vi "CIGrab.vi"(8 "Camera data":variant, 9 "TrackingParameters":T1={"Corner-based bead pos (out)"=[], "QTrk Instance"={"QTrk Pointer"=0}, "Tracking Config"={"Number of steps"=0, "ZLUT stepsize (um)"=0.0, "Z correction factor"=0.0, "Start piezo Z (um)"=0.0, "Pixel size (nm)"=0.0, "2D Localization Type"=enum."Quadrant Interpolation", "Z Command (None)"=enum."Nothing"}, "ResultManager"={"InstancePtr"=0}, "Send to queue?"=TRUE}, 10 "Output Queue":refnum<queue>, 11 "GrabControlQueue":refnum<queue>) -> (0 "Camera (out)":variant)   [LabVIEW 2011]
uses:
  BeadTracker2.llb/CmdData_NewFrame.ctl
  <vilib>/vision/Image Controls.llb/IMAQ Image.ctl
  BeadTracker2.llb/CmdEnum_CameraFrameType.ctl
  BeadTracker2.llb/CIGrabParams.ctl
  qtrk/QTrk.llb/QTrkInstance.ctl
  BeadTracker2.llb/TrackingConfigType.ctl
  qtrk/QTrk.llb/QTrkLocalizationType.ctl
  qtrk/QTrk.llb/QTrkZCommandType.ctl
  qtrk/QTrk.llb/ResultManagerInstance.ctl
  BeadTracker2.llb/CIGrabControlMsg.ctl
  BeadTracker2.llb/CIGrabControlMsgEnum.ctl
  mkCameraData.ctl
  CameraConfig.ctl
  BeadTracker2.llb/GenericCameraConfigType.ctl
panel:
  in  "Check ROIs":bool
  out "Status Information : Lost Frames":u32
  in  "Tracking enabled?":bool
  in  "stop":bool
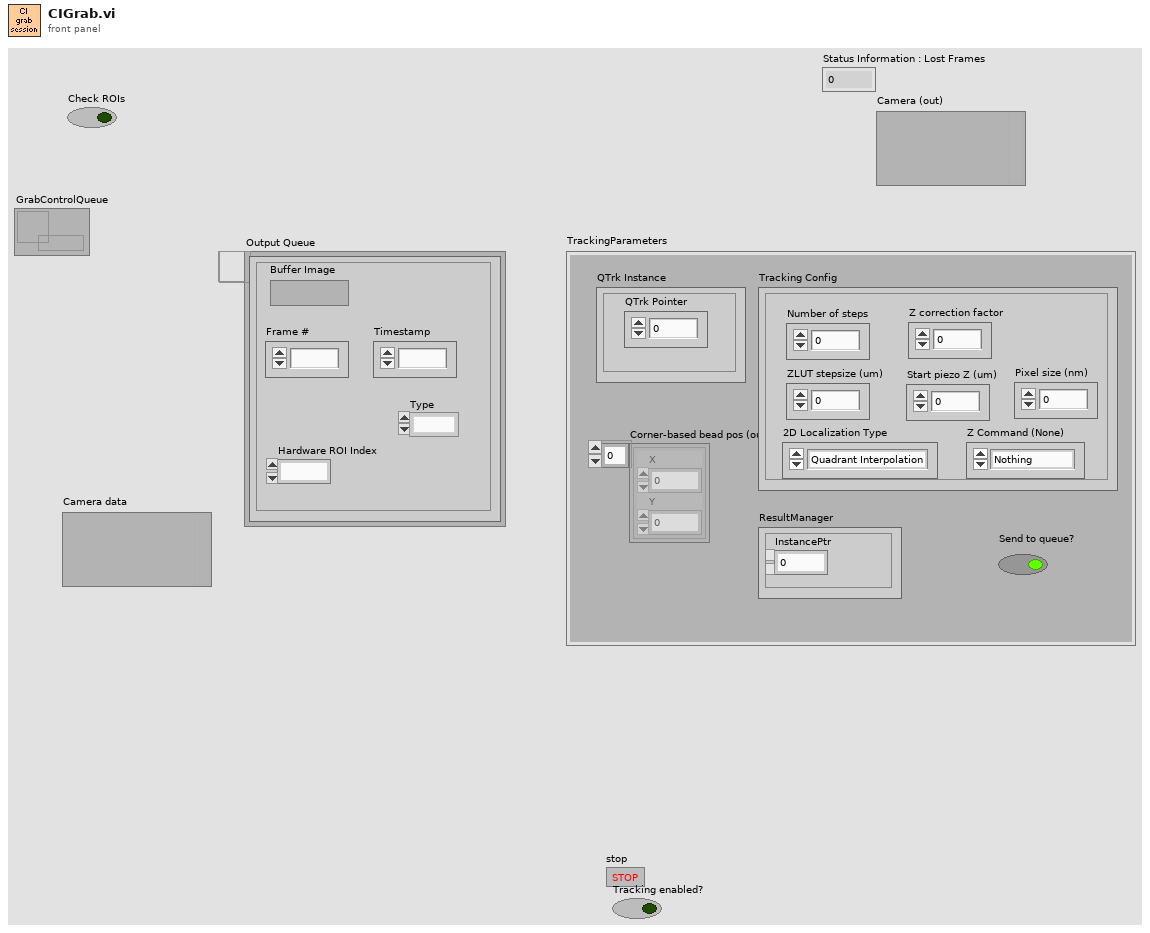
[diagram p1: front panel]
types:
  T1 = typedef "CIGrabParams.ctl" = cluster{"Corner-based bead pos (out)":cluster{"X":i32, "Y":i32}[], "QTrk Instance":T2, "Tracking Config":T3, "ResultManager":T6, "Send to queue?":bool}
  T2 = typedef "QTrkInstance.ctl" = cluster{"QTrk Pointer":u64}
  T3 = typedef "TrackingConfigType.ctl" = cluster{"Number of steps":i32, "ZLUT stepsize (um)":sgl, "Z correction factor":sgl, "Start piezo Z (um)":sgl, "Pixel size (nm)":sgl, "2D Localization Type":T4, "Z Command (None)":T5}
  T4 = typedef "QTrkLocalizationType.ctl" = enum16{"Center-of-Mass", "1D Cross-Correlation", "Quadrant Interpolation", "Gaussian 2D MLE"}
  T5 = typedef "QTrkZCommandType.ctl" = enum16{"Nothing", "ComputeZ", "BuildRadialZLUT", "BuildImageZLUT", "RadialZLUT+ImageZLUT"}
  T6 = typedef "ResultManagerInstance.ctl" = cluster{"InstancePtr":u64}
  T7 = typedef "mkCameraData.ctl" = cluster{"Session":refnum<k11>, "Settings":T8}
  T8 = typedef "CameraConfig.ctl" = cluster{"Gain [1-4]":sgl, "Offset":i16, "Mode":i16, "ROIs":cluster{"X":i32, "Y":i32}[], "ROI Size":cluster{"X":i32, "Y":i32}, "Number of buffers":i32, "Use hardware multiple-ROI?":bool, "GenericCameraConfig":T9}
  T9 = typedef "GenericCameraConfigType.ctl" = cluster{"Framerate (Hz)":i32, "Exposure time (us)":i32, "Image size":cluster{"Width":i32, "Height":i32}}
  T10 = typedef "QTrkComputedSettings.ctl" = cluster{"QTrk Settings":T11, "Derived settings":cluster{"ZLUT Radial Steps":i32, "ZLUT Angular Steps":i32, "ZLUT Max Radius":sgl, "QI Radial Steps":i32, "QI Angular Steps\nPer Quadrant":i32, "QI Max Radius":sgl}}
  T11 = typedef "QTrkSettings.ctl" = cluster{"Image width":i32, "Image height":i32, "Number of threads (CPU based)":i32, "CUDA Device":i32, "COM Background correction factor":sgl, "ZLUT MinRadius":sgl, "ZLUT Radial sample density":sgl, "ZLUT Angular sample density":sgl, "ZLUT ROI Coverage":sgl, "QI Iterations":i32, "QI MinRadius":sgl, "QI Radial sample density":sgl, "QI Angular sample density":sgl, "QI ROI Coverage":sgl, "QI Angular Step \nIteration Factor":sgl, "XCOR Profile Length":i32, "XCOR Profile Width":i32, "XCOR Iterations":i32, "Gaussian 2D Fit Iterations":i32, "Gaussian 2D Sigma (pixels)":sgl}
  T12 = typedef "CIGrabControlMsg.ctl" = cluster{"Msg":T13}
  T13 = typedef "CIGrabControlMsgEnum.ctl" = enum16{"Stop", "EnableTracking", "DisableTracking"}
  T14 = typedef "CmdEnum_CameraFrameType.ctl" = enum16{"Full", "HardwareROI", "EndGrabMarker"}
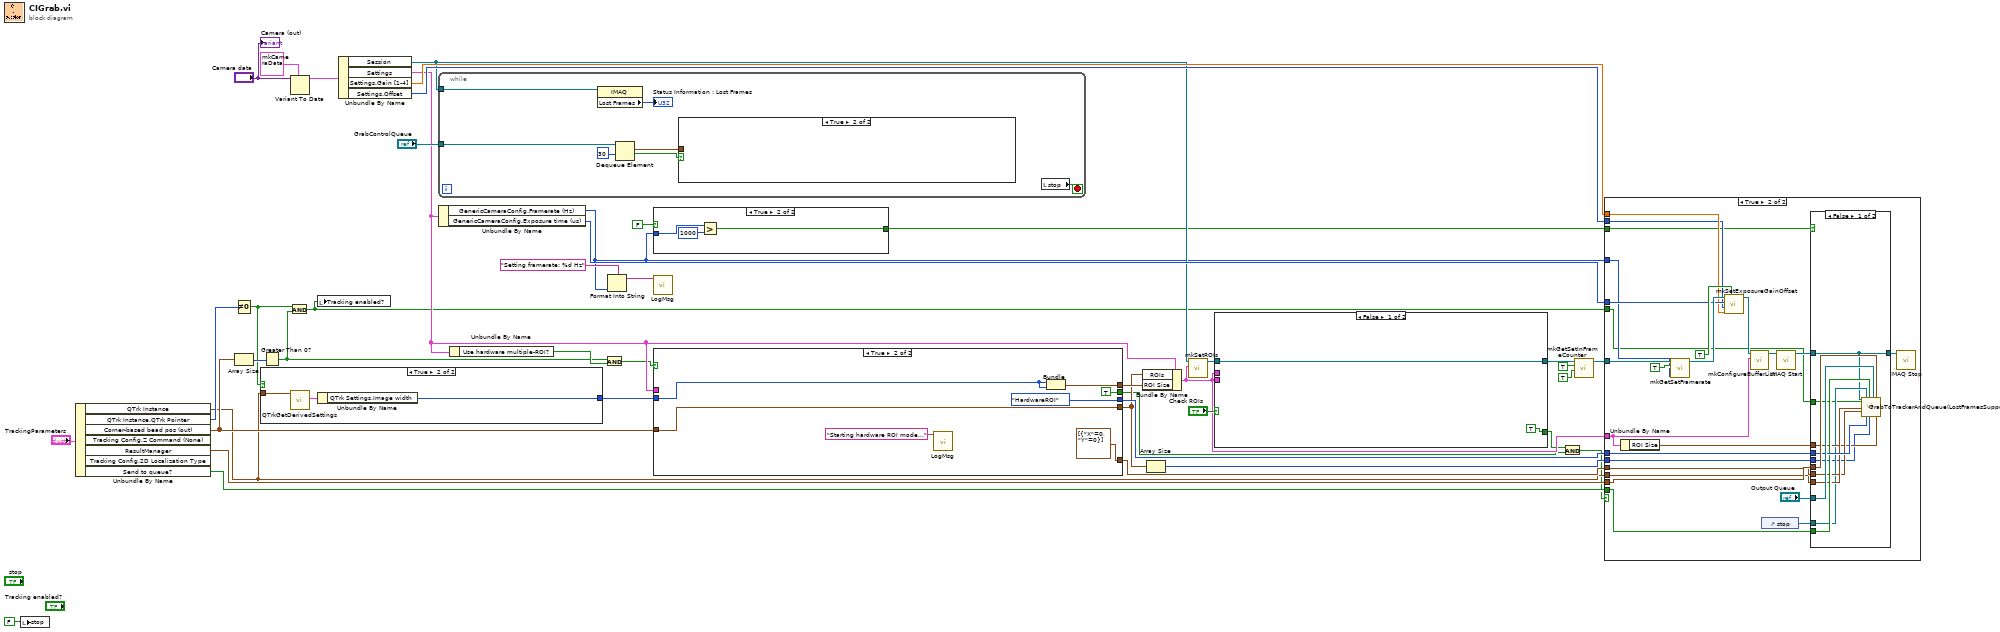
[diagram p0: block diagram]
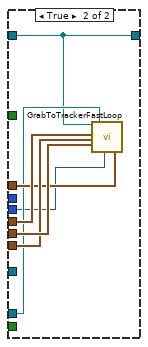
[diagram p3: hidden frame]
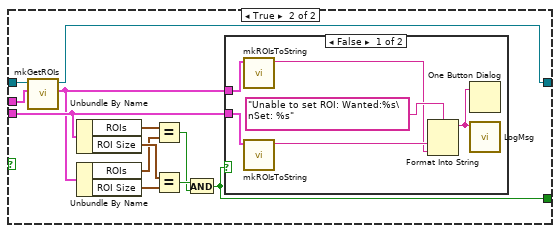
[diagram p4: hidden frame]
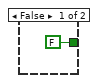
[diagram p6: hidden frame]
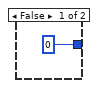
[diagram p7: hidden frame]
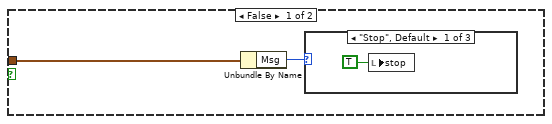
[diagram p8: hidden frame]
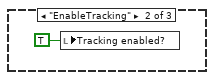
[diagram p9: hidden frame]
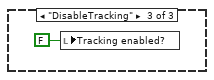
[diagram p10: hidden frame]
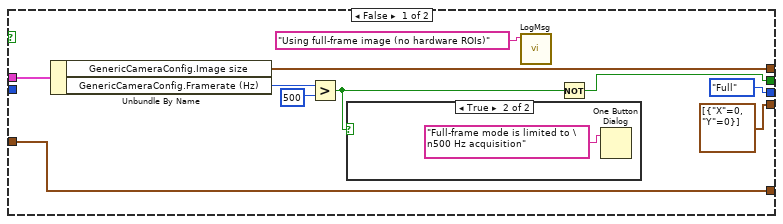
[diagram p11: hidden frame]
diagram:
  n1 = local write "stop"(FALSE ("stop")) -> ()
  n2 = Unbundle By Name("TrackingParameters") -> ("QTrk Instance"=w15:T2, "QTrk Instance.QTrk Pointer"=w37:u64, "Corner-based bead pos (out)"=w31:cluster{"X":i32, "Y":i32}[], "ResultManager"=w35:T6, "Send to queue?"=w27:bool)  [unwired: 2 out]
  n3 = Not Equal To 0?(x=w37) -> (x != 0?=w16:bool)
  n4 = Array Size(array=w31) -> (size(s)=w30:i32)
  n5 = case shown="True" w16 {
    tunnel: w15 -> [_ w46]
    tunnel: [0 ("Image width") w45] -> w14
    frame False {
    }
    frame True {
      n6 = call "QTrkGetDerivedSettings.vi"("QTrk Instance"=w46) -> ("Derived settings"=w47:T10)  [unwired: 5 in, 5 out]
      n7 = Unbundle By Name(w47) -> ("QTrk Settings.Image width"=w45:i32)
    }
  }
  n8 = Greater Than 0?(x=w30) -> (x > 0?=w28:bool)
  n9 = Variant To Data(type=T7 {"Session"=refnum, "Settings"={"Gain [1-4]"=1.0, "Offset"=50, "Mode"=6, "ROIs"=[], "ROI Size"={"X"=0, "Y"=0}, "Number of buffers"=40, "Use hardware multiple-ROI?"=FALSE, "GenericCameraConfig"={"Framerate (Hz)"=0, "Exposure time (us)"=0, "Image size"={"Width"=0, "Height"=0}}}} ("Camera data"), Variant="Camera data") -> (data=w8:T7)  [unwired: 1 in, 1 out]
  n10 = And(x=w16, y=w28) -> (x .and. y?=w10:bool)
  n11 = local write "Tracking enabled?"(w10) -> ()
  n12 = Unbundle By Name(w8) -> ("Session"=w26:refnum<k11>, "Settings"=w22:T8, "Settings.Gain [1-4]"=w39:sgl, "Settings.Offset"=w38:i16)
  n13 = while {
    tunnel: "GrabControlQueue" -> [w54]
    tunnel: w26 -> [w49]
    stop <- w51 stop-if-true
    n14 = property class="IMAQ"(reference=w49) -> ("Lost Frames"=→"Status Information : Lost Frames":u32)  [unwired: 1 in, 2 out]
    n15 = Dequeue Element(queue=w54, timeout in ms (-1)=30) -> (element=w52:T12, timed out?=w53:bool)  [unwired: 1 in, 2 out]
    n16 = case shown="True" w53 {
      tunnel: w52 -> [w56 _]
      frame False {
        n17 = Unbundle By Name(w56) -> ("Msg"=w55:T13)
        n18 = case shown="\"Stop\", Default" w55 {
          frame "Stop", Default {
            n19 = local write "stop"(TRUE ("stop")) -> ()
          }
          frame "EnableTracking" {
            n20 = local write "Tracking enabled?"(TRUE ("Tracking enabled?")) -> ()
          }
          frame "DisableTracking" {
            n21 = local write "Tracking enabled?"(FALSE ("Tracking enabled?")) -> ()
          }
        }
      }
      frame True {
      }
    }
    n22 = local read "stop"() -> (w51:bool)
  }
  n23 = Unbundle By Name(w22) -> ("GenericCameraConfig.Framerate (Hz)"=w13:i32, "GenericCameraConfig.Exposure time (us)"=w40:i32)
  n24 = Unbundle By Name(w22) -> ("Use hardware multiple-ROI?"=w29:bool)
  n25 = And(x=w28, y=w29) -> (x .and. y?=w17:bool)
  n26 = Format Into String(format string="Setting framerate: %d Hz", w13) -> (resulting string=w25:string)  [unwired: 2 in, 1 out]
  n27 = case shown="True" FALSE {
    tunnel: w13 -> [_ w63]
    tunnel: [FALSE w61] -> w12
    frame False {
    }
    frame True {
      n28 = Greater?(x=w63, y=1000) -> (0:w61:bool)
    }
  }
  n29 = call "LogMsg.vi"("msg"=w25) -> ()  [unwired: 11 in]
  n30 = case shown="True" w17 {
    tunnel: [w71 w81] -> w36
    tunnel: w31 -> [w69 w77]
    tunnel: [cluster{"X":i32, "Y":i32}[] [{"X"=0, "Y"=0}] ("ROIs") w77] -> w21
    tunnel: [CmdEnum_CameraFrameType."Full" ("Type") CmdEnum_CameraFrameType."HardwareROI" ("Type")] -> w33
    tunnel: w22 -> [w72 _]
    tunnel: [w69 cluster{"X":i32, "Y":i32}[] [{"X"=0, "Y"=0}] ("ROIs")] -> w23
    tunnel: w14 -> [_ w76]
    tunnel: [w64 TRUE] -> w1
    frame False {
      n31 = Unbundle By Name(w72) -> ("GenericCameraConfig.Image size"=w71:cluster{"Width":i32, "Height":i32}, "GenericCameraConfig.Framerate (Hz)"=w67:i32)
      n32 = Greater?(x=w67, y=500) -> (0:w65:bool)
      n33 = case shown="True" w65 {
        frame False {
        }
        frame True {
          n34 = One Button Dialog(message="Full-frame mode is limited to \n500 Hz acquisition") -> ()  [unwired: 1 in, 1 out]
        }
      }
      n35 = call "LogMsg.vi"("msg"="Using full-frame image (no hardware ROIs)") -> ()  [unwired: 11 in]
      n36 = Not(x=w65) -> (.not. x?=w64:bool)
    }
    frame True {
      n37 = call "LogMsg.vi"("msg"="Starting hardware ROI mode...") -> ()  [unwired: 11 in]
      n38 = Bundle("Image width"=w76, "Image width"=w76) -> (w81:cluster{"Image width":i32, "Image width":i32})  [unwired: 1 in]
    }
  }
  n39 = Bundle By Name(cluster=w22, "ROIs"=w21, "ROI Size"=w36) -> (w4:T8)
  n40 = Array Size(array=w21) -> (size(s)=w18:i32)
  n41 = call "mkSetROIs.vi"("Camera in"=w4, "IMAQ Refnum in"=w26) -> ("IMAQ Refnum out"=w7:refnum<k11>)  [unwired: 9 in]
  n42 = case shown="False" "Check ROIs" {
    tunnel: w7 -> [w83 w95]
    tunnel: w4 -> [_ w94]
    tunnel: [w83 w93] -> w6
    tunnel: w4 -> [_ w85]
    tunnel: [TRUE w88] -> w3
    frame False {
    }
    frame True {
      n43 = call "mkGetROIs.vi"("Camera settings"=w94, "IMAQ Refnum in"=w95) -> ("Camera settings (out)"=w84:T8, "IMAQ Refnum out"=w93:refnum<k11>)  [unwired: 8 in]
      n44 = Unbundle By Name(w85) -> ("ROIs"=w92:cluster{"X":i32, "Y":i32}[], "ROI Size"=w91:cluster{"X":i32, "Y":i32})
      n45 = Unbundle By Name(w84) -> ("ROIs"=w86:cluster{"X":i32, "Y":i32}[], "ROI Size"=w87:cluster{"X":i32, "Y":i32})
      n46 = Equal?(x=w92, y=w86) -> (x = y?=w89:bool)
      n47 = Equal?(x=w91, y=w87) -> (x = y?=w90:bool)
      n48 = And(x=w90, y=w89) -> (x .and. y?=w88:bool)
      n49 = case shown="False" w88 {
        tunnel: w85 -> [w99 _]
        tunnel: w84 -> [w98 _]
        frame False {
          n50 = call "mkROIsToString.vi"("Settings"=w98) -> ("ROIs description"=w97:string)  [unwired: 10 in]
          n51 = call "mkROIsToString.vi"("Settings"=w99) -> ("ROIs description"=w100:string)  [unwired: 10 in]
          n52 = Format Into String(format string="Unable to set ROI: Wanted:%s\nSet: %s", w100, w97) -> (resulting string=w96:string)  [unwired: 2 in, 1 out]
          n53 = One Button Dialog(message=w96) -> ()  [unwired: 1 in, 1 out]
          n54 = call "LogMsg.vi"("msg"=w96) -> ()  [unwired: 11 in]
        }
        frame True {
        }
      }
    }
  }
  n55 = And(x=w3, y=w1) -> (x .and. y?=w2:bool)
  n56 = call "mkGetSetInFrameCounter.vi"("Set? (F)"=TRUE, "Enable in-frame counter (T)"=TRUE, "IMAQ Refnum in"=w6) -> ("IMAQ Refnum out"=w20:refnum<k11>)  [unwired: 7 in, 1 out]
  n57 = case shown="True" w2 {
    tunnel: w40 -> [_ w118]
    tunnel: w39 -> [_ w117]
    tunnel: w38 -> [_ w116]
    tunnel: w35 -> [_ w115]
    tunnel: w33 -> [_ w114]
    tunnel: w27 -> [_ w113]
    tunnel: w23 -> [_ w112]
    tunnel: w20 -> [_ w111]
    tunnel: w18 -> [_ w109]
    tunnel: w15 -> [_ w107]
    tunnel: w13 -> [_ w106]
    tunnel: w12 -> [_ w105]
    tunnel: w10 -> [_ w103]
    tunnel: w4 -> [_ w102]
    frame False {
    }
    frame True {
      n58 = Unbundle By Name(w102) -> ("ROI Size"=w108:cluster{"X":i32, "Y":i32})
      n59 = call "mkGetSetFramerate.vi"("Framerate"=w106, "Set? (F)"=TRUE, "IMAQ Refnum out"=w111) -> ("IMAQ Refnum (out)"=w123:refnum<k11>)  [unwired: 5 in, 3 out]
      n60 = call "mkSetExposureGainOffset.vi"("Set? (F)"=TRUE, "Gain [1-4]"=w117, "Offset"=w116, "Exposure time"=w118, "IMAQ Refnum in"=w123) -> ("IMAQ Refnum out"=w122:refnum<k11>)  [unwired: 1 in, 5 out]
      n61 = call "mkConfigureBufferList.vi"("Camera in"=w102, "IMAQ Session"=w122) -> ("IMAQ Session (out)"=w120:refnum<k11>)  [unwired: 9 in]
      n62 = control-ref of="stop"() -> (w104:refnum<vi>)
      n63 = call <vilib>:"IMAQ Start.vi"("IMAQ Session In"=w120) -> ("IMAQ Session Out"=w110:refnum<k11>)  [unwired: 9 in, 1 out]
      n64 = case shown="False" w105 {
        tunnel: "Output Queue" -> [w136 _]
        tunnel: w115 -> [w135 w143]
        tunnel: w114 -> [w134 _]
        tunnel: w113 -> [w133 _]
        tunnel: w107 -> [w132 w141]
        tunnel: w112 -> [w131 w142]
        tunnel: w108 -> [w130 w140]
        tunnel: w104 -> [w129 w139]
        tunnel: w103 -> [w128 _]
        tunnel: w109 -> [w127 w138]
        tunnel: w110 -> [w126 w137]
        tunnel: [w126 w137] -> w121
        frame False {
          n65 = call "GrabToTrackerAndQueue(LostFramesSupport).vi"("IMAQ Refnum in"=w126, "Tracking enabled?"=w128, "QTrk Instance"=w132, "ROIs"=w131, "stop"=w129, "Type"=w134, "Send to queue?"=w133, "#ROI"=w127, "Output Queue"=w136, "ResultManager"=w135, "ROI Size"=w130) -> ()  [unwired: 9 in]
        }
        frame True {
          n66 = call "GrabToTrackerFastLoop.vi"("IMAQ Refnum in"=w137, "ResultManager"=w143, "QTrk Instance"=w141, "ROIs"=w142, "stop"=w139, "#ROI"=w138, "ROI Size"=w140) -> ()  [unwired: 13 in]
        }
      }
      n67 = call <vilib>:"IMAQ Stop.vi"("IMAQ Session In"=w121) -> ()  [unwired: 9 in, 2 out]
    }
  }
  "Camera (out)" <- "Camera data"
